vi "create error message.vi"(8 "error in (no error)":errorcluster, 11 "queues":T1) -> ()   [LabVIEW 2018]
uses:
  type defs/Queues.ctl
  supporting VIs/polymorphic VIs/enqueue for comms.vi
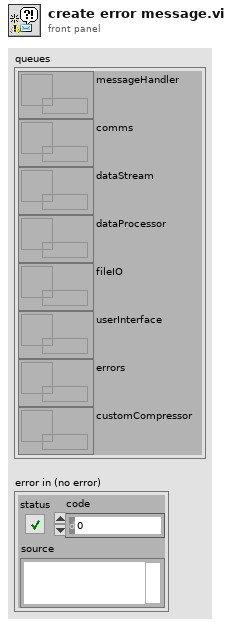
[diagram p1: front panel]
types:
  T1 = typedef "Queues.ctl" = cluster{"messageHandler":refnum<queue>, "comms":refnum<queue>, "dataStream":refnum<queue>, "dataProcessor":refnum<queue>, "fileIO":refnum<queue>, "userInterface":refnum<queue>, "errors":refnum<queue>, "customCompressor":refnum<queue>}
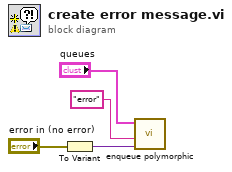
[diagram p0: block diagram]
diagram:
  n1 = To Variant(anything="error in (no error)") -> (Variant=w1:variant)
  n2 = call-poly "enqueue polymorphic.vi"("data"=w1, "message"="error", "Queues"="queues") -> ()  [unwired: 8 in, 1 out]
